vi "Write Value.vi"(8 "error in (no error)":errorcluster, 10 "Value":u64, 11 "fixed64 in":refnum<class "fixed64.lvclass">) -> (0 "error out":errorcluster, 3 "fixed64 out":refnum<class "fixed64.lvclass">)   [LabVIEW 2020, in "Protobuf RAW.lvlib" / "fixed64.lvclass"]
uses:
  fixed64.lvclass
  fixed64.lvclass/fixed64.ctl
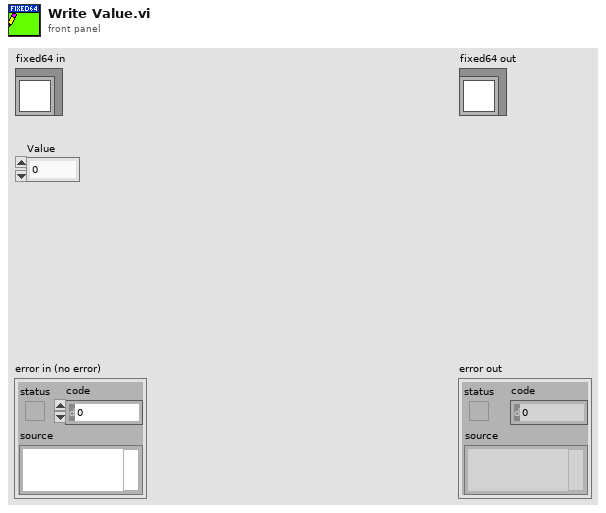
[diagram p1: front panel]
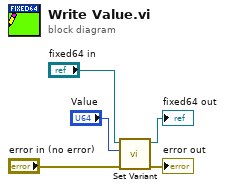
[diagram p0: block diagram]
diagram:
  n1 = call-dynamic "Set Variant.vi"("error in (no error)"="error in (no error)", "Value"="Value", "Proto Type Common in"="fixed64 in") -> ("error out"=→"error out":errorcluster, "Proto Type Common out"=→"fixed64 out":refnum<class "fixed64.lvclass">)  [unwired: 7 in]
